vi "OAT Round to Nearest Boundary.vi"(2 "x in":dbl format="%.2f", 3 "boundary":dbl format="%.2f") -> (4 "x out":dbl format="%.2f")   [LabVIEW 2017]
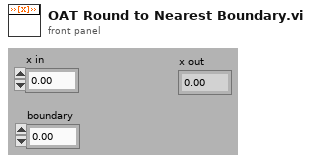
[diagram p1: front panel]
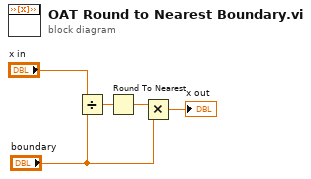
[diagram p0: block diagram]
diagram:
  n1 = Divide(x="x in", y="boundary") -> (x/y=w4:dbl)
  n2 = Round To Nearest(number=w4) -> (nearest integer value=w3:dbl)
  n3 = Multiply(x=w3, y="boundary") -> (x*y=→"x out":dbl)
